vi "gxml_EscapeChars.vi"(10 "XML In":string) -> (2 "XML Out":string)   [LabVIEW 2011, in "Third Party VIs.lvlib" / "GXML.lvlib"]
doc: "This VI escapes all characters with decimal codes between 128 and 255 to &#nnn; (nnn is the decimal code)"
uses:
  GXML.lvlib
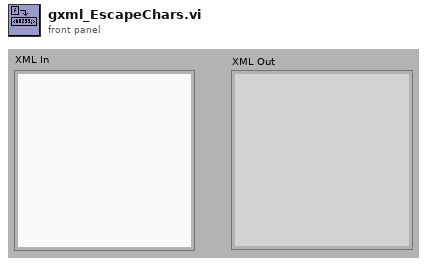
[diagram p1: front panel]
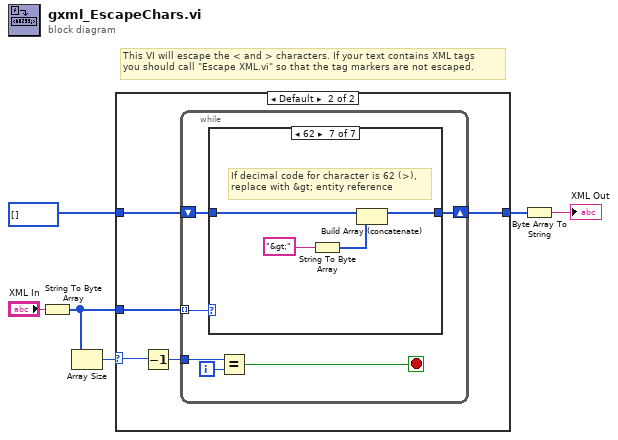
[diagram p0: block diagram]
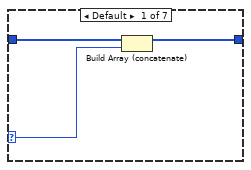
[diagram p3: hidden frame]
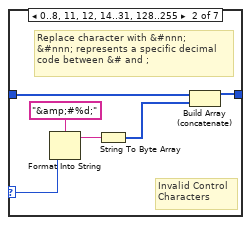
[diagram p4: hidden frame]
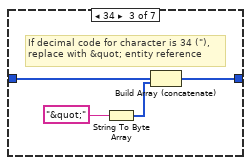
[diagram p5: hidden frame]
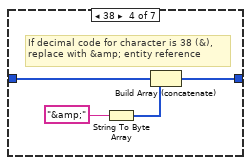
[diagram p6: hidden frame]
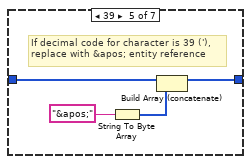
[diagram p7: hidden frame]
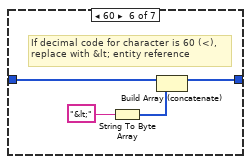
[diagram p8: hidden frame]
diagram:
  # "This VI will escape the < and > characters. If your text contains XML tags\nyou should call \"Escape XML.vi\" so that the tag markers are not escaped."
  n1 = String To Byte Array(string="XML In") -> (unsigned byte array=w5:u8[])
  n2 = Array Size(array=w5) -> (size(s)=w1:i32)
  n3 = case shown="Default" w1 {
    selector: w1 -> [_ w8]
    tunnel: u8[] [] -> [_ w12]
    tunnel: w5 -> [w7 w11]
    tunnel: [w7 w9] -> w4
    frame 0 {
    }
    frame Default {
      n4 = Decrement(x=w8) -> (x-1=w10:i32)
      n5 = while {
        tunnel: w11 -> [w15] mode=indexing
        shift-right: [w17] -> w9
        shift-left: w12 -> [w18]
        tunnel: w10 -> [w14]
        i -> [w16]
        stop <- w13 stop-if-true
        n6 = case shown="62" w15 {
          selector: w15 -> [w19 w23 _ _ _ _ _]
          tunnel: w18 -> [w21 w27 w30 w34 w37 w41 w45]
          tunnel: [w20 w26 w29 w33 w36 w40 w44] -> w17
          frame Default {
            n7 = Build Array (concatenate)(w21, w19) -> (w20:u8[])
          }
          frame 0..8, 11, 12, 14..31, 128..255 {
            # "Invalid Control\nCharacters"
            # "Replace character with &#nnn;\n&#nnn; represents a specific decimal\ncode between &# and ;"
            n8 = Format Into String(format string="&amp;#%d;" ("Format String"), w23) -> (resulting string=w25:string)  [unwired: 2 in, 1 out]
            n9 = String To Byte Array(string=w25) -> (unsigned byte array=w24:u8[])
            n10 = Build Array (concatenate)(w27, w24) -> (w26:u8[])
          }
          frame 34 {
            # "If decimal code for character is 34 (\"),\nreplace with &quot; entity reference"
            n11 = String To Byte Array(string="&quot;" ("Format String")) -> (unsigned byte array=w28:u8[])
            n12 = Build Array (concatenate)(w30, w28) -> (w29:u8[])
          }
          frame 38 {
            # "If decimal code for character is 38 (&),\nreplace with &amp; entity reference"
            n13 = String To Byte Array(string="&amp;" ("Format String")) -> (unsigned byte array=w32:u8[])
            n14 = Build Array (concatenate)(w34, w32) -> (w33:u8[])
          }
          frame 39 {
            # "If decimal code for character is 39 ('),\nreplace with &apos; entity reference"
            n15 = String To Byte Array(string="&apos;" ("Format String")) -> (unsigned byte array=w38:u8[])
            n16 = Build Array (concatenate)(w37, w38) -> (w36:u8[])
          }
          frame 60 {
            # "If decimal code for character is 60 (<),\nreplace with &lt; entity reference"
            n17 = String To Byte Array(string="&lt;" ("Format String")) -> (unsigned byte array=w42:u8[])
            n18 = Build Array (concatenate)(w41, w42) -> (w40:u8[])
          }
          frame 62 {
            # "If decimal code for character is 62 (>),\nreplace with &gt; entity reference"
            n19 = String To Byte Array(string="&gt;" ("Format String")) -> (unsigned byte array=w46:u8[])
            n20 = Build Array (concatenate)(w45, w46) -> (w44:u8[])
          }
        }
        n21 = Equal?(x=w14, y=w16) -> (x = y?=w13:bool)
      }
    }
  }
  n22 = Byte Array To String(unsigned byte array=w4) -> (string=→"XML Out":string)
